vi "DC Magnet On.vi"(7 "Shutdown Delay (2 s)":dbl[unit]=2.0 format="%.1f", 8 "error in":errorcluster, 9 "Current Compliance Level (400 mA)":dbl[unit]=0.4 step=0.01 format="%.1f", 10 "Pulse Duration (10 s)":dbl[unit]=10.0 format="%.1f", 11 "VISA resource name":refnum<visa-resource-name>="GPIB0::6::INSTR") -> (0 "error out":errorcluster, 1 "SMU Current AFTER Shutdown Duration (mA)":sgl=-1.0 format="%#_5f", 2 "SMU Current BEFORE Shutdown Duration (mA)":sgl=-1.0 format="%#_5f", 3 "VISA resource dup":refnum<visa-resource-name>)   [LabVIEW 2010]
doc: "This function pulses a DC electromagnet using the Keithley 24xx SMU as a current source."
uses:
  <instrlib>/Keithley 24XX/Public/Data/Read (Single Point).vi
  <instrlib>/Keithley 24XX/Keithley 24XX.lvlib
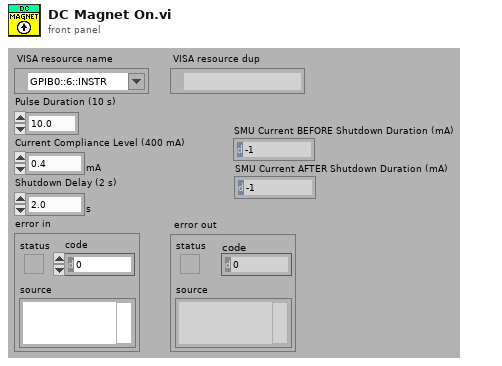
[diagram p1: front panel]
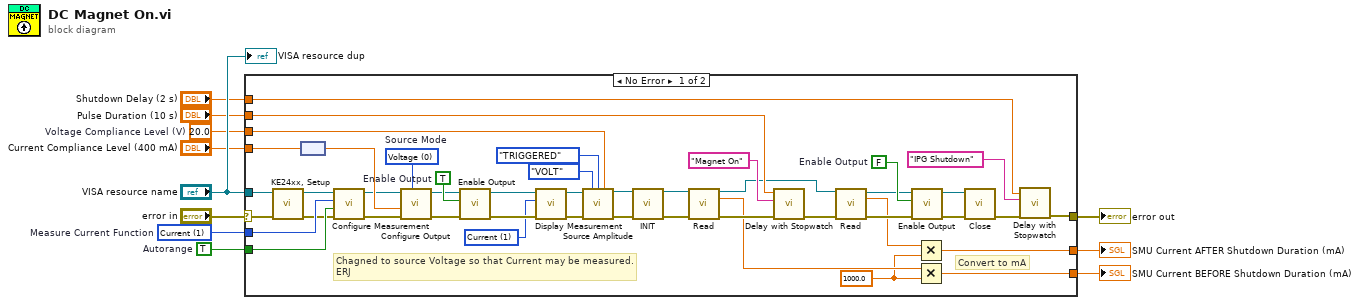
[diagram p0: block diagram]
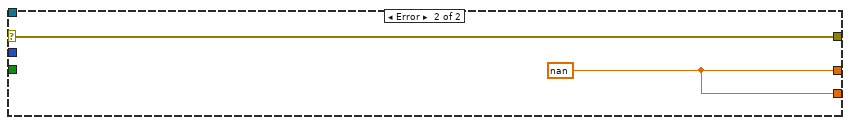
[diagram p2: hidden frame]
diagram:
  w10 = TRUE  # Autorange
  w8 = u16 1 items=["Volts", "Current", "Resistance"]  # Measure Current Function
  w4 = 20.0  # Voltage Compliance Level (V)
  n1 = case shown="No Error" "error in" {
    selector: "error in" -> [w51 w58]
    tunnel: [w40 w58] -> w11
    tunnel: w4 -> [w29 _]
    tunnel: "VISA resource name" -> [w50 _]
    tunnel: w10 -> [w55 _]
    tunnel: w8 -> [w56 _]
    tunnel: "Current Compliance Level (400 mA)" -> [w52 _]
    tunnel: "Pulse Duration (10 s)" -> [w45 _]
    tunnel: "Shutdown Delay (2 s)" -> [w38 _]
    tunnel: [w12 w57] -> w1
    tunnel: [w13 w57] -> w2
    frame No Error {
      w14 = sgl 1000.0 ("y")
      w23 = TRUE  # Enable Output
      w24 = u16 1 items=["Voltage", "Current", "Resistance"] ("Displayed Measurement (0: Voltage)")
      w44 = FALSE  # Enable Output
      w49 = u16 0 items=["Voltage", "Current"]  # Source Mode
      # "Convert to mA"
      # "Chagned to source Voltage so that Current may be measured.\nERJ"
      n2 = call "KE24xx, Setup.vi"("error in"=w51, "VISA rsrc"=w50) -> ("error out"=w21:errorcluster, "VISA rsrc out"=w22:refnum<visa-resource-name>)  [unwired: 6 in]
      n3 = node(w52) -> (w30:dbl)
      n4 = call <instrlib>:"Configure Measurement.vi"("error in (no error)"=w21, "Enable Auto Range (T:Enable)"=w55, "Function (0: Volts)"=w56, "VISA resource name"=w22) -> ("error out"=w19:errorcluster, "VISA resource name out"=w20:refnum<visa-resource-name>)  [unwired: 6 in]
      n5 = call <instrlib>:"Configure Output.vi"("Source Mode  (0: Voltage)"=w49, "error in (no error)"=w19, "Compliance  Level (0.1)"=w30, "VISA resource name"=w20) -> ("error out"=w18:errorcluster, "VISA resource name out"=w17:refnum<visa-resource-name>)  [unwired: 6 in]
      n6 = call <instrlib>:"Enable Output.vi"("error in (no error)"=w18, "Enable Output (T: Enable)"=w23, "VISA resource name"=w17) -> ("error out"=w28:errorcluster, "VISA resource name out"=w26:refnum<visa-resource-name>)  [unwired: 7 in]
      n7 = call <instrlib>:"Display Measurement.vi"("error in (no error)"=w28, "Displayed Measurement (0: Voltage)"=w24, "VISA resource name"=w26) -> ("error out"=w27:errorcluster, "VISA resource name out"=w25:refnum<visa-resource-name>)  [unwired: 7 in]
      n8 = call "Source Amplitude.vi"("VISA resource name"=w25, "Source Function"=enum16{"CURR", "VOLT"}."VOLT", "Mode"=enum16{"IMM", "TRIGGERED"}."TRIGGERED", "Source Level"=w29, "error in (no error)"=w27) -> ("VISA resource name out"=w48:refnum<visa-resource-name>, "error out"=w47:errorcluster)  [unwired: 9 in]
      n9 = call "INIT.vi"("VISA resource name"=w48, "error in (no error)"=w47) -> ("VISA resource name out"=w37:refnum<visa-resource-name>, "error out"=w36:errorcluster)  [unwired: 12 in]
      n10 = call-poly <instrlib>:"Read.vi"("VISA resource name"=w37, "error in (no error)"=w36) -> ("VISA resource name out"=w31:refnum<visa-resource-name>, "Current"=w15:sgl, "error out"=w35:errorcluster)  [unwired: 7 in, 4 out]
      n11 = call "Delay with Stopwatch.vi"("error in"=w35, "window title"="Magnet On", "delay"=w45) -> ("error out"=w34:errorcluster)  [unwired: 4 in]
      n12 = call-poly <instrlib>:"Read.vi"("VISA resource name"=w31, "error in (no error)"=w34) -> ("VISA resource name out"=w32:refnum<visa-resource-name>, "Current"=w16:sgl, "error out"=w33:errorcluster)  [unwired: 7 in, 4 out]
      n13 = call <instrlib>:"Enable Output.vi"("error in (no error)"=w33, "Enable Output (T: Enable)"=w44, "VISA resource name"=w32) -> ("error out"=w43:errorcluster, "VISA resource name out"=w42:refnum<visa-resource-name>)  [unwired: 7 in]
      n14 = Multiply(x=w16, y=w14) -> (x*y=w13:sgl)
      n15 = Multiply(x=w15, y=w14) -> (x*y=w12:sgl)
      n16 = call <instrlib>:"Close.vi"("error in (no error)"=w43, "VISA resource name"=w42) -> ("error out"=w41:errorcluster)  [unwired: 9 in]
      n17 = call "Delay with Stopwatch.vi"("error in"=w41, "window title"="IPG Shutdown", "delay"=w38) -> ("error out"=w40:errorcluster)  [unwired: 4 in]
    }
    frame Error {
      w57 = sgl nan
    }
  }
  "error out" <- w11
  "SMU Current BEFORE Shutdown Duration (mA)" <- w1
  "SMU Current AFTER Shutdown Duration (mA)" <- w2
  "VISA resource dup" <- "VISA resource name"
